vi "montaCabecalho.vi"(0 "addr":u8=15 format="%.0b", 11 "opcode":u8=15 format="%.0b") -> (8 "Cabeçalho":u8 format="%.0x")   [LabVIEW 2018]
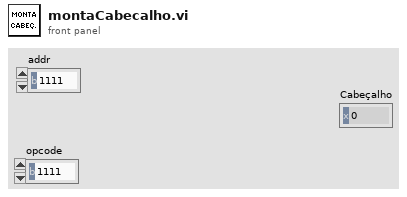
[diagram p1: front panel]
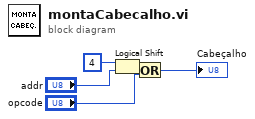
[diagram p0: block diagram]
diagram:
  n1 = Logical Shift(y=u16 4, x="addr") -> (x << y=w2:u8)
  n2 = Or(x=w2, y="opcode") -> (x .or. y?=→"Cabeçalho":u8)
